vi "Write U32 FIFO - 4 spc.vi"(0 "input data":u32[](array[numeric])=[0, 0, 0, 0], 1 "reset":bool, 2 "fifo":refnum<k21>, 9 "input valid":bool) -> (14 "ready for input":bool)   [LabVIEW 2023]
uses:
  <vilib>/rvi/DataTransferAndStorage/Container/Common/niFpgaContainerExecOnDevCompGetState.vi
  <vilib>/rvi/Emulation/niFpgaSctlEmulationGetInTimedLoop.vi
  <vilib>/rvi/errors/niFpgaSetErrorForExecOnDevCompSimple.vi
  <vilib>/rvi/eio/common/nirviEmuReportErrorAndStop.vi
  <vilib>/rvi/interface/RandomDataEmulation/nirviRandomDataAcquireLock.vi
  <vilib>/rvi/interface/RandomDataEmulation/nirviRandomDataQueueStore.vi
  <vilib>/rvi/interface/RandomDataEmulation/nirviRandomDataReleaseLock.vi
  <vilib>/rvi/interface/RandomDataEmulation/nirviFPGAContextMergeError.vi
  <vilib>/rvi/interface/RandomDataEmulation/nirviRandomDataCheckExitLoopConditions.vi
  <vilib>/express/rvi/timingcommon/nirviCommon.vi
  <vilib>/rvi/interface/RandomDataEmulation/niFpgaRandomDataHandleErrors.vi
  <vilib>/rvi/DataTransferAndStorage/Container/XNode/niFpgaContainer.xnode
  <vilib>/rvi/FIFO/Fifo_Resource/niFpgaFifoEmulationRefInMultiElement.vi
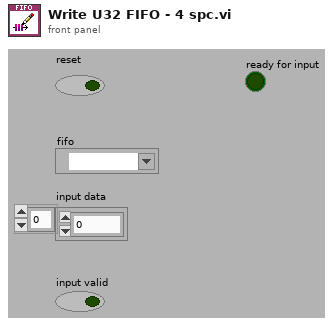
[diagram p1: front panel]
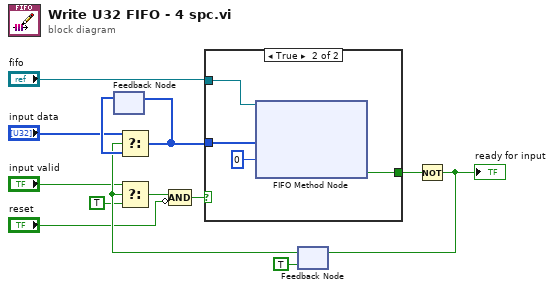
[diagram p0: block diagram]
diagram:
  n1 = feedback #1() -> (w12:u32[])  [unwired: 1 in]
  n2 = feedback #2(TRUE) -> (w10:bool)
  n3 = Select(t="input data", s=w10, f=w12) -> (s? t:f=w11:u32[])
  n4 = feedback-in #1(w11) -> ()
  n5 = Select(t="input valid", s=w10, f=TRUE) -> (s? t:f=w6:bool)
  n6 = Compound Arithmetic op=AND(w6, invert "reset") -> (w4:bool)
  n7 = case shown="True" w4 {
    tunnel: "fifo" -> [_ w17]
    tunnel: w11 -> [_ w15]
    tunnel: [_ w14] -> w3
    frame False {
    }
    frame True {
      n8 = xnode ("FIFO Method Node")("Element"=w15, "Timeout"=0, "FIFO In"=w17) -> ("Timed Out?"=w14:bool)  [unwired: 1 out]
    }
  }
  n9 = Not(x=w3) -> (.not. x?=w2:bool)
  "ready for input" <- w2
  n10 = feedback-in #2(w2) -> ()
